vi "GRA_SAPER_RUN.vi"() -> ()   [LabVIEW 2021]
panel:
  out "flag":bool
  out "Czas gry":dbl format="%<%M:%S>t"
  out ".not. x?":bool
  out "Miny":i32
  out "resta":i32
  out "mat17":i32[][](array[numeric])
  out "rozmiar":i32
  in  "cluster3":T1
  in  "Cluster 2":T2
  in  "Cluster 1":T3
  out "licznik":i32[][](array[numeric])
  out "miny":i32[][](array[numeric])
  out "zdjecia":i32[][](array[ring])
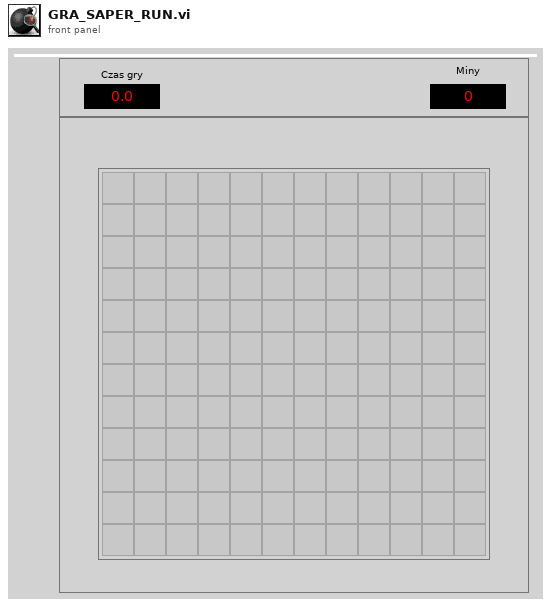
[diagram p1: front panel]
types:
  T1 = cluster{"Boolean 65":bool, "Boolean 66":bool, "Boolean 67":bool, "Boolean 68":bool, "Boolean 69":bool, "Boolean 70":bool, "Boolean 71":bool, "Boolean 72":bool, "Boolean 73":bool, "Boolean 74":bool, "Boolean 75":bool, "Boolean 76":bool, "Boolean 77":bool, "Boolean 78":bool, "Boolean 79":bool, "Boolean 80":bool, "Boolean 81":bool, "Boolean 82":bool, "Boolean 83":bool, "Boolean 84":bool, "Boolean 85":bool, "Boolean 86":bool, "Boolean 87":bool, "Boolean 88":bool, "Boolean 89":bool, "Boolean 90":bool, "Boolean 91":bool, "Boolean 92":bool, "Boolean 93":bool, "Boolean 94":bool, "Boolean 95":bool, "Boolean 96":bool, "Boolean 97":bool, "Boolean 98":bool, "Boolean 99":bool, "Boolean 100":bool, "Boolean 101":bool, "Boolean 102":bool, "Boolean 103":bool, "Boolean 104":bool, "Boolean 105":bool, "Boolean 106":bool, "Boolean 107":bool, "Boolean 108":bool, "Boolean 109":bool, "Boolean 110":bool, "Boolean 111":bool, "Boolean 112":bool, "Boolean 113":bool, "Boolean 114":bool, "Boolean 115":bool, "Boolean 116":bool, "Boolean 117":bool, "Boolean 118":bool, "Boolean 119":bool, "Boolean 120":bool, "Boolean 121":bool, "Boolean 122":bool, "Boolean 123":bool, "Boolean 124":bool, "Boolean 125":bool, "Boolean 126":bool, "Boolean 127":bool, "Boolean 128":bool, "Boolean 129":bool, "Boolean 130":bool, "Boolean 131":bool, "Boolean 132":bool, "Boolean 133":bool, "Boolean 134":bool, "Boolean 135":bool, "Boolean 136":bool, "Boolean 137":bool, "Boolean 138":bool, "Boolean 139":bool, "Boolean 140":bool, "Boolean 141":bool, "Boolean 142":bool, "Boolean 143":bool, "Boolean 144":bool, "Boolean 145":bool, "Boolean 146":bool, "Boolean 147":bool, "Boolean 148":bool, "Boolean 149":bool, "Boolean 150":bool, "Boolean 151":bool, "Boolean 152":bool, "Boolean 153":bool, "Boolean 154":bool, "Boolean 155":bool, "Boolean 156":bool, "Boolean 157":bool, "Boolean 158":bool, "Boolean 159":bool, "Boolean 160":bool, "Boolean 161":bool, "Boolean 162":bool, "Boolean 163":bool, "Boolean 164":bool, "Boolean 165":bool, "Boolean 166":bool, "Boolean 167":bool, "Boolean 168":bool, "Boolean 169":bool, "Boolean 170":bool, "Boolean 171":bool, "Boolean 172":bool, "Boolean 173":bool, "Boolean 174":bool, "Boolean 175":bool, "Boolean 176":bool, "Boolean 177":bool, "Boolean 178":bool, "Boolean 179":bool, "Boolean 180":bool, "Boolean 181":bool, "Boolean 182":bool, "Boolean 183":bool, "Boolean 184":bool, "Boolean 185":bool, "Boolean 186":bool, "Boolean 187":bool, "Boolean 188":bool, "Boolean 189":bool, "Boolean 190":bool, "Boolean 191":bool, "Boolean 192":bool, "Boolean 193":bool, "Boolean 194":bool, "Boolean 195":bool, "Boolean 196":bool, "Boolean 197":bool, "Boolean 198":bool, "Boolean 199":bool, "Boolean 200":bool, "Boolean 201":bool, "Boolean 202":bool, "Boolean 203":bool, "Boolean 204":bool, "Boolean 205":bool, "Boolean 206":bool, "Boolean 207":bool, "Boolean 208":bool}
  T2 = cluster{"Boolean 65":bool, "Boolean 66":bool, "Boolean 67":bool, "Boolean 68":bool, "Boolean 69":bool, "Boolean 70":bool, "Boolean 71":bool, "Boolean 72":bool, "Boolean 77":bool, "Boolean 78":bool, "Boolean 79":bool, "Boolean 80":bool, "Boolean 81":bool, "Boolean 82":bool, "Boolean 83":bool, "Boolean 84":bool, "Boolean 89":bool, "Boolean 90":bool, "Boolean 91":bool, "Boolean 92":bool, "Boolean 93":bool, "Boolean 94":bool, "Boolean 95":bool, "Boolean 96":bool, "Boolean 101":bool, "Boolean 102":bool, "Boolean 103":bool, "Boolean 104":bool, "Boolean 105":bool, "Boolean 106":bool, "Boolean 107":bool, "Boolean 108":bool, "Boolean 113":bool, "Boolean 114":bool, "Boolean 115":bool, "Boolean 116":bool, "Boolean 117":bool, "Boolean 118":bool, "Boolean 119":bool, "Boolean 120":bool, "Boolean 125":bool, "Boolean 126":bool, "Boolean 127":bool, "Boolean 128":bool, "Boolean 129":bool, "Boolean 130":bool, "Boolean 131":bool, "Boolean 132":bool, "Boolean 137":bool, "Boolean 138":bool, "Boolean 139":bool, "Boolean 140":bool, "Boolean 141":bool, "Boolean 142":bool, "Boolean 143":bool, "Boolean 144":bool, "Boolean 149":bool, "Boolean 150":bool, "Boolean 151":bool, "Boolean 152":bool, "Boolean 153":bool, "Boolean 154":bool, "Boolean 155":bool, "Boolean 156":bool}
  T3 = cluster{"Boolean 65":bool, "Boolean 66":bool, "Boolean 67":bool, "Boolean 68":bool, "Boolean 69":bool, "Boolean 70":bool, "Boolean 77":bool, "Boolean 78":bool, "Boolean 79":bool, "Boolean 80":bool, "Boolean 81":bool, "Boolean 82":bool, "Boolean 89":bool, "Boolean 90":bool, "Boolean 91":bool, "Boolean 92":bool, "Boolean 93":bool, "Boolean 94":bool, "Boolean 101":bool, "Boolean 102":bool, "Boolean 103":bool, "Boolean 104":bool, "Boolean 105":bool, "Boolean 106":bool, "Boolean 113":bool, "Boolean 114":bool, "Boolean 115":bool, "Boolean 116":bool, "Boolean 117":bool, "Boolean 118":bool, "Boolean 125":bool, "Boolean 126":bool, "Boolean 127":bool, "Boolean 128":bool, "Boolean 129":bool, "Boolean 130":bool}
  T4 = cluster{"Boolean 6":bool, "Boolean 6":bool, "Boolean 7":bool, "Boolean 8":bool, "Boolean 9":bool, "Boolean 10":bool, "Boolean 11":bool, "Boolean 12":bool, "Boolean 13":bool, "Boolean 14":bool, "Boolean 15":bool, "Boolean 16":bool, "Boolean 17":bool, "Boolean 18":bool, "Boolean 19":bool, "Boolean 20":bool, "Boolean 21":bool, "Boolean 22":bool, "Boolean 23":bool, "Boolean 24":bool, "Boolean 25":bool, "Boolean 26":bool, "Boolean 27":bool, "Boolean 28":bool, "Boolean 29":bool, "Boolean 30":bool, "Boolean 31":bool, "Boolean 32":bool, "Boolean 33":bool, "Boolean 34":bool, "Boolean 35":bool, "Boolean 36":bool, "Boolean 37":bool, "Boolean 38":bool, "Boolean 39":bool, "Boolean 40":bool, "Boolean 41":bool, "Boolean 42":bool, "Boolean 43":bool, "Boolean 44":bool, "Boolean 45":bool, "Boolean 46":bool, "Boolean 47":bool, "Boolean 48":bool, "Boolean 49":bool, "Boolean 50":bool, "Boolean 51":bool, "Boolean 52":bool, "Boolean 53":bool, "Boolean 54":bool, "Boolean 55":bool, "Boolean 56":bool, "Boolean 57":bool, "Boolean 58":bool, "Boolean 59":bool, "Boolean 60":bool, "Boolean 61":bool, "Boolean 62":bool, "Boolean 63":bool, "Boolean 64":bool, "Boolean 65":bool, "Boolean 66":bool, "Boolean 67":bool, "Boolean 68":bool, "Boolean 69":bool, "Boolean 70":bool, "Boolean 71":bool, "Boolean 72":bool, "Boolean 73":bool, "Boolean 74":bool, "Boolean 75":bool, "Boolean 76":bool, "Boolean 77":bool, "Boolean 78":bool, "Boolean 79":bool, "Boolean 80":bool, "Boolean 81":bool, "Boolean 82":bool, "Boolean 83":bool, "Boolean 84":bool, "Boolean 85":bool, "Boolean 86":bool, "Boolean 87":bool, "Boolean 88":bool, "Boolean 89":bool, "Boolean 90":bool, "Boolean 91":bool, "Boolean 92":bool, "Boolean 93":bool, "Boolean 94":bool, "Boolean 95":bool, "Boolean 96":bool, "Boolean 97":bool, "Boolean 98":bool, "Boolean 99":bool, "Boolean 100":bool, "Boolean 101":bool, "Boolean 102":bool, "Boolean 103":bool, "Boolean 104":bool, "Boolean 105":bool, "Boolean 106":bool, "Boolean 107":bool, "Boolean 108":bool, "Boolean 109":bool, "Boolean 110":bool, "Boolean 111":bool, "Boolean 112":bool, "Boolean 113":bool, "Boolean 114":bool, "Boolean 115":bool, "Boolean 116":bool, "Boolean 117":bool, "Boolean 118":bool, "Boolean 119":bool, "Boolean 120":bool, "Boolean 121":bool, "Boolean 122":bool, "Boolean 123":bool, "Boolean 124":bool, "Boolean 125":bool, "Boolean 126":bool, "Boolean 127":bool, "Boolean 128":bool, "Boolean 129":bool, "Boolean 130":bool, "Boolean 131":bool, "Boolean 132":bool, "Boolean 133":bool, "Boolean 134":bool, "Boolean 135":bool, "Boolean 136":bool, "Boolean 137":bool, "Boolean 138":bool, "Boolean 139":bool, "Boolean 140":bool, "Boolean 141":bool, "Boolean 142":bool, "Boolean 143":bool, "Boolean 144":bool, "Boolean 145":bool, "Boolean 146":bool, "Boolean 147":bool, "Boolean 148":bool}
  T5 = cluster{"Boolean 6":bool, "Boolean 6":bool, "Boolean 7":bool, "Boolean 8":bool, "Boolean 9":bool, "Boolean 10":bool, "Boolean 11":bool, "Boolean 12":bool, "Boolean 17":bool, "Boolean 18":bool, "Boolean 19":bool, "Boolean 20":bool, "Boolean 21":bool, "Boolean 22":bool, "Boolean 23":bool, "Boolean 24":bool, "Boolean 29":bool, "Boolean 30":bool, "Boolean 31":bool, "Boolean 32":bool, "Boolean 33":bool, "Boolean 34":bool, "Boolean 35":bool, "Boolean 36":bool, "Boolean 41":bool, "Boolean 42":bool, "Boolean 43":bool, "Boolean 44":bool, "Boolean 45":bool, "Boolean 46":bool, "Boolean 47":bool, "Boolean 48":bool, "Boolean 53":bool, "Boolean 54":bool, "Boolean 55":bool, "Boolean 56":bool, "Boolean 57":bool, "Boolean 58":bool, "Boolean 59":bool, "Boolean 60":bool, "Boolean 65":bool, "Boolean 66":bool, "Boolean 67":bool, "Boolean 68":bool, "Boolean 69":bool, "Boolean 70":bool, "Boolean 71":bool, "Boolean 72":bool, "Boolean 77":bool, "Boolean 78":bool, "Boolean 79":bool, "Boolean 80":bool, "Boolean 81":bool, "Boolean 82":bool, "Boolean 83":bool, "Boolean 84":bool, "Boolean 89":bool, "Boolean 90":bool, "Boolean 91":bool, "Boolean 92":bool, "Boolean 93":bool, "Boolean 94":bool, "Boolean 95":bool, "Boolean 96":bool}
  T6 = cluster{"Boolean 6":bool, "Boolean 6":bool, "Boolean 7":bool, "Boolean 8":bool, "Boolean 9":bool, "Boolean 10":bool, "Boolean 17":bool, "Boolean 18":bool, "Boolean 19":bool, "Boolean 20":bool, "Boolean 21":bool, "Boolean 22":bool, "Boolean 29":bool, "Boolean 30":bool, "Boolean 31":bool, "Boolean 32":bool, "Boolean 33":bool, "Boolean 34":bool, "Boolean 41":bool, "Boolean 42":bool, "Boolean 43":bool, "Boolean 44":bool, "Boolean 45":bool, "Boolean 46":bool, "Boolean 53":bool, "Boolean 54":bool, "Boolean 55":bool, "Boolean 56":bool, "Boolean 57":bool, "Boolean 58":bool, "Boolean 65":bool, "Boolean 66":bool, "Boolean 67":bool, "Boolean 68":bool, "Boolean 69":bool, "Boolean 70":bool}
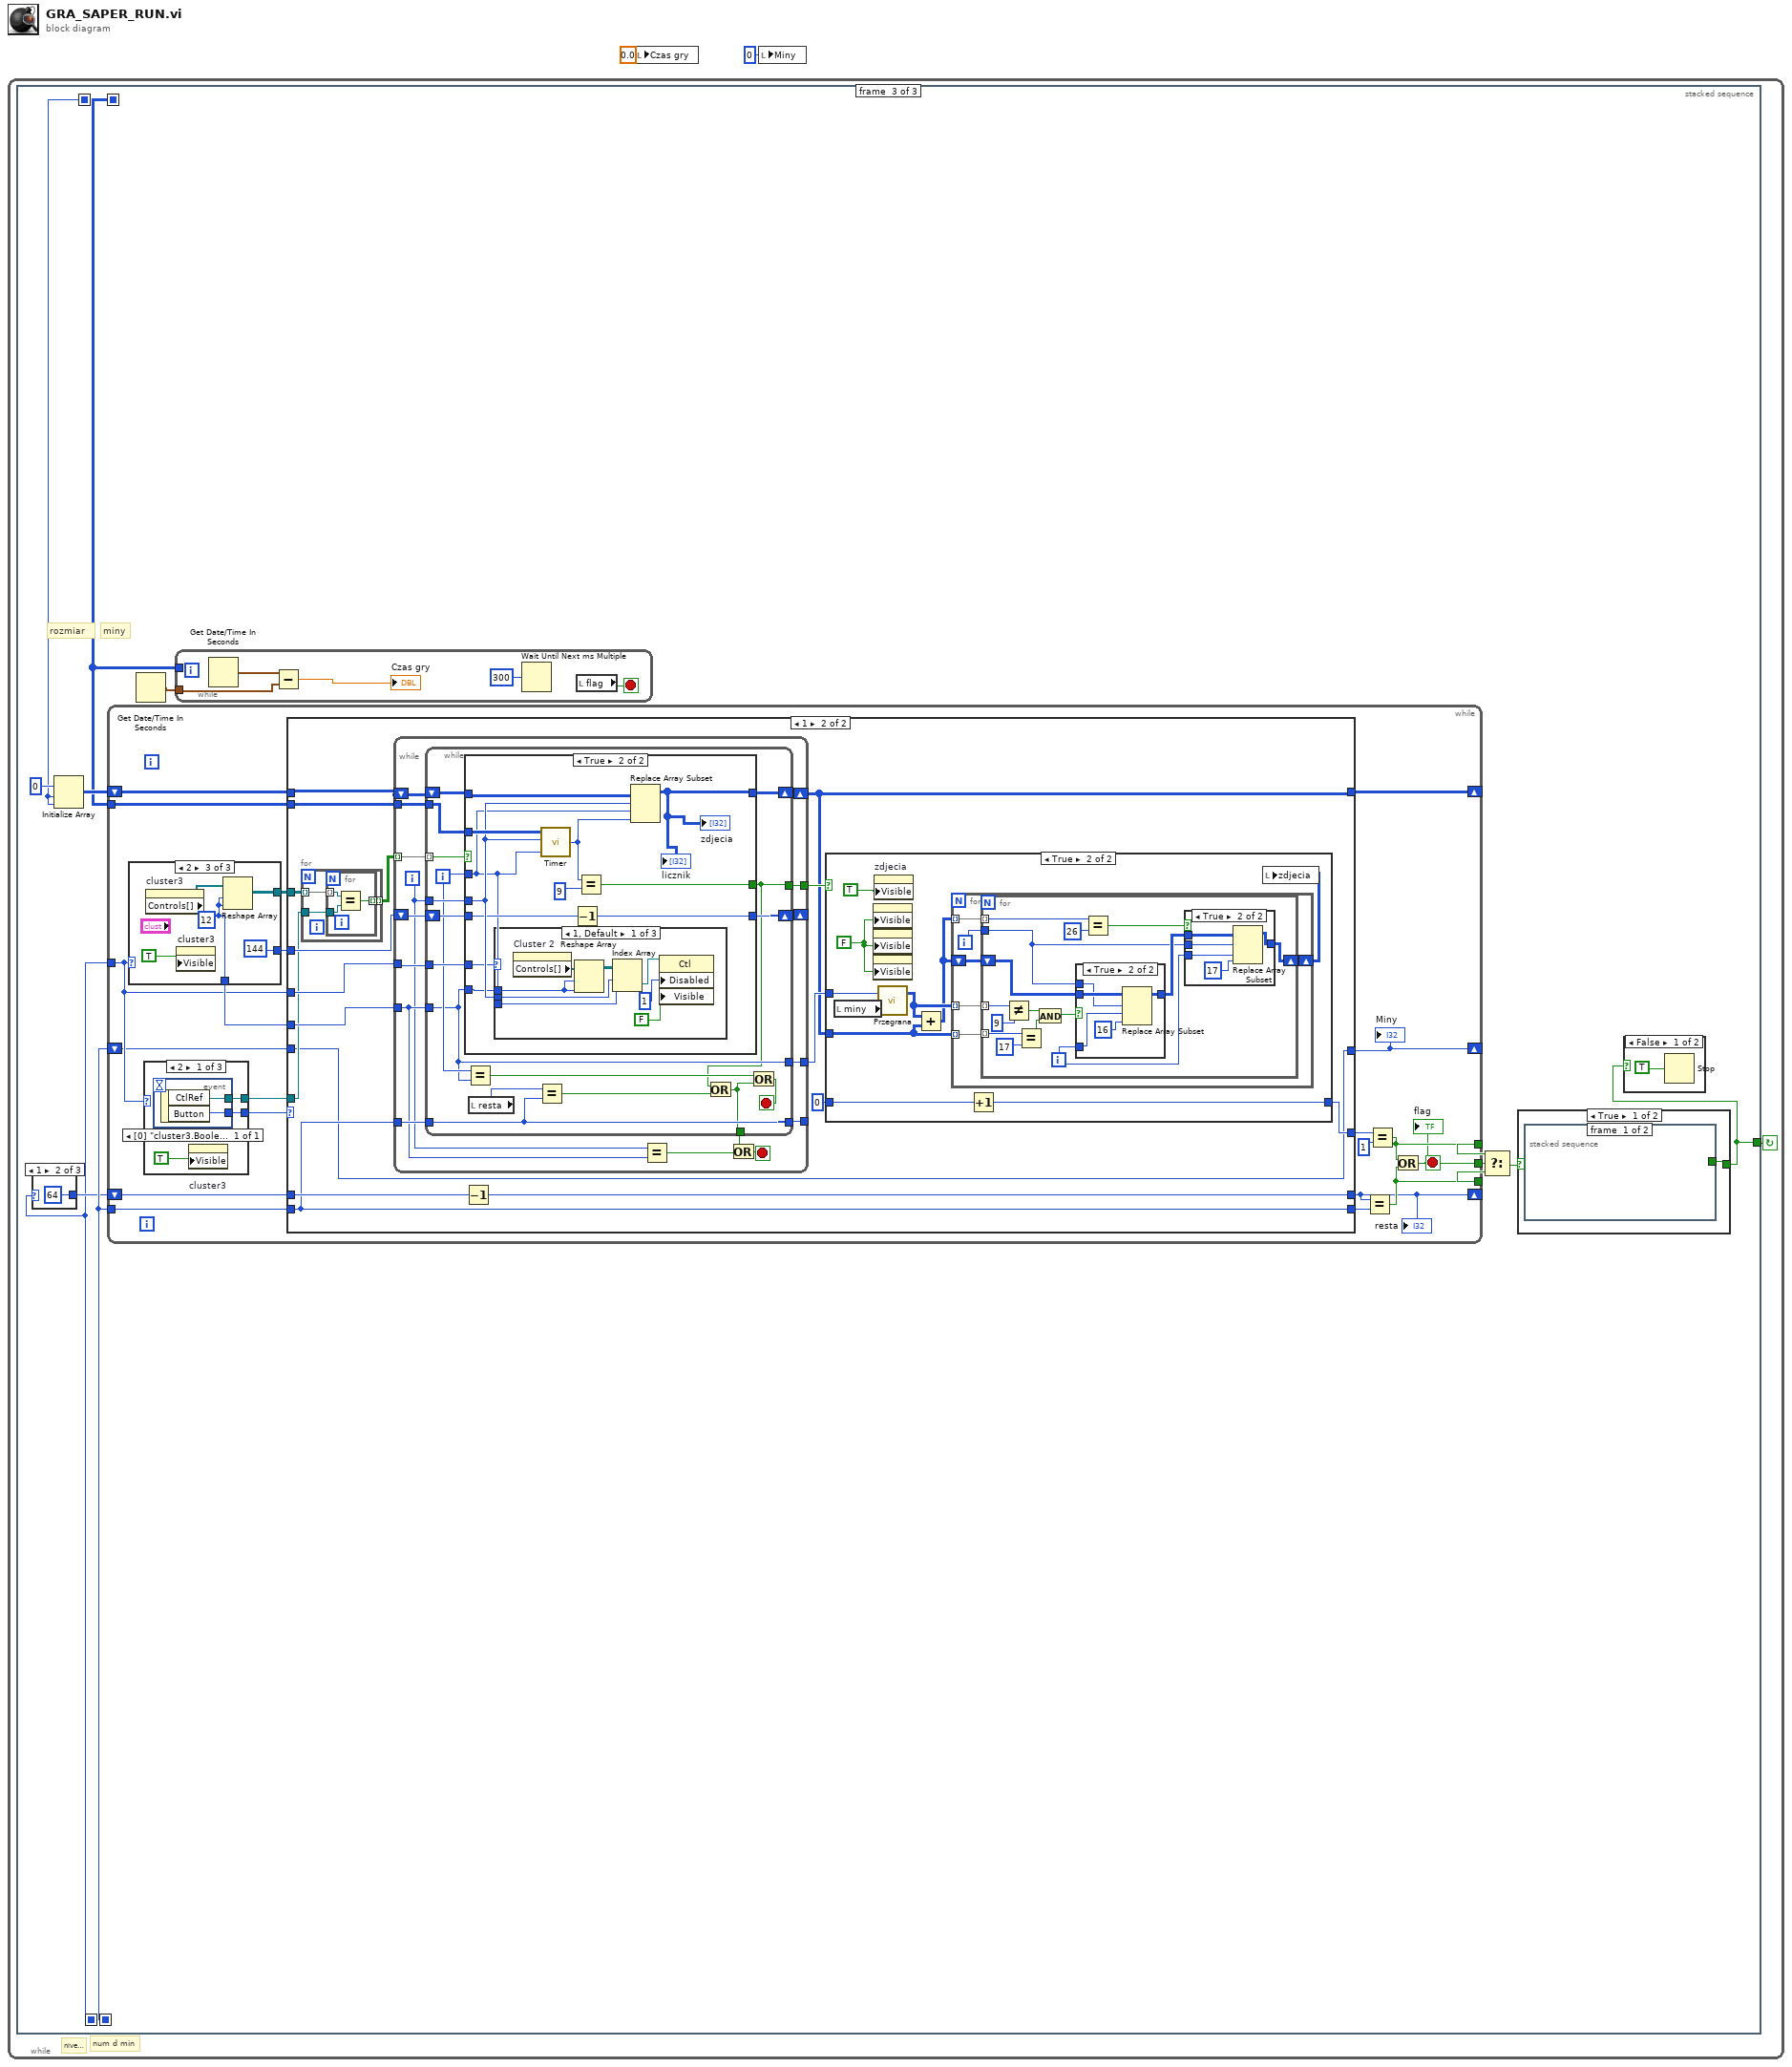
[diagram p0: block diagram]
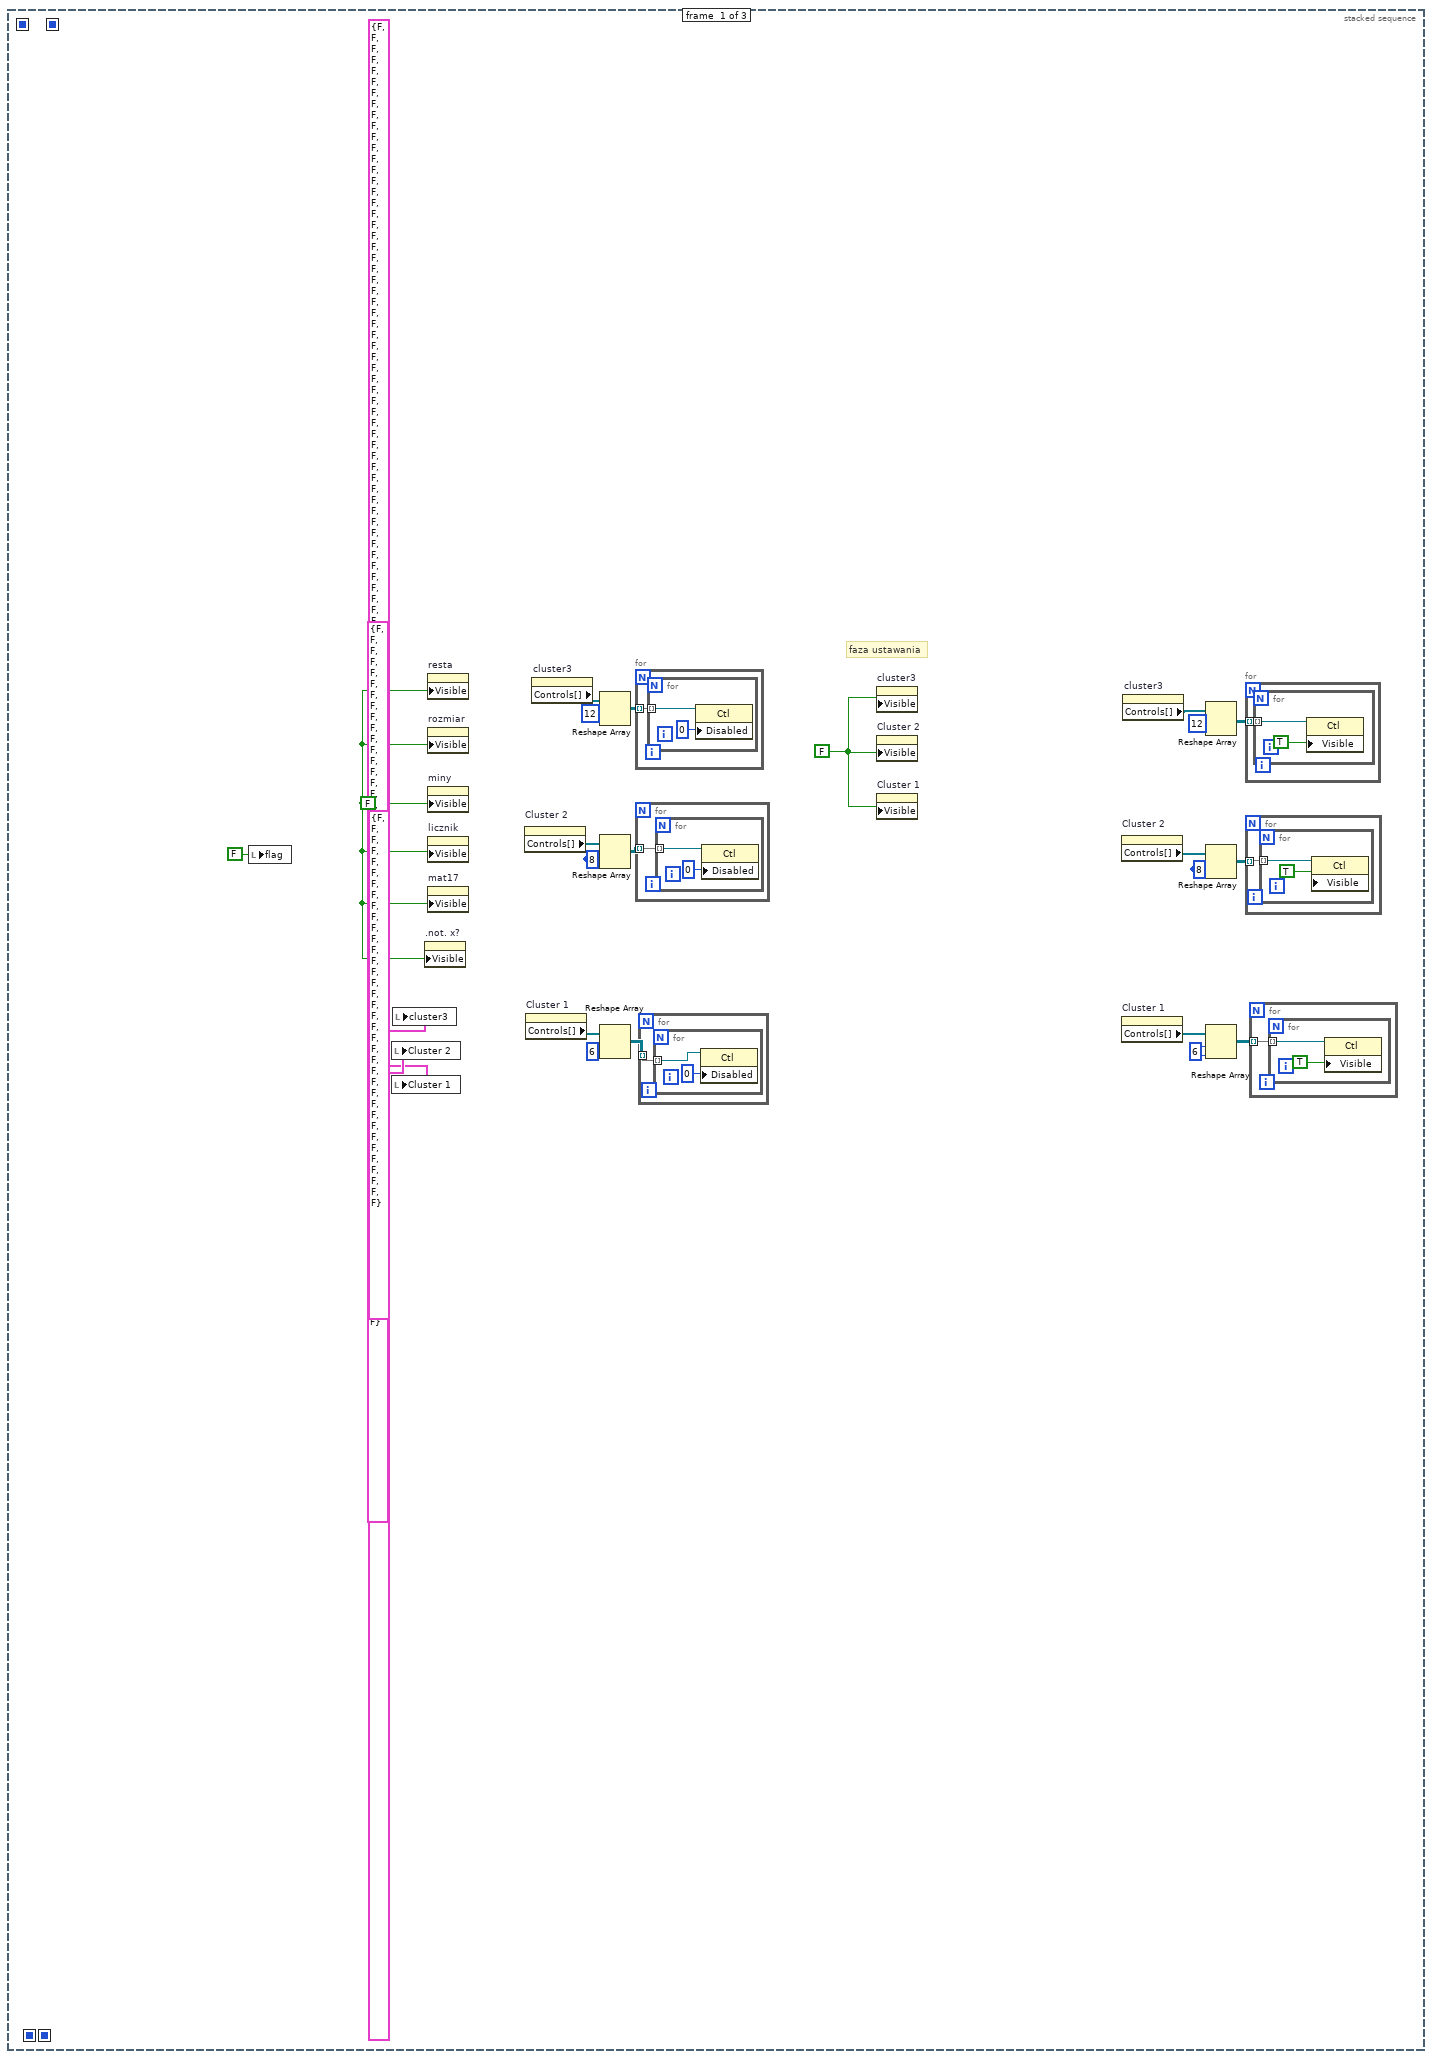
[diagram p2: hidden frame]
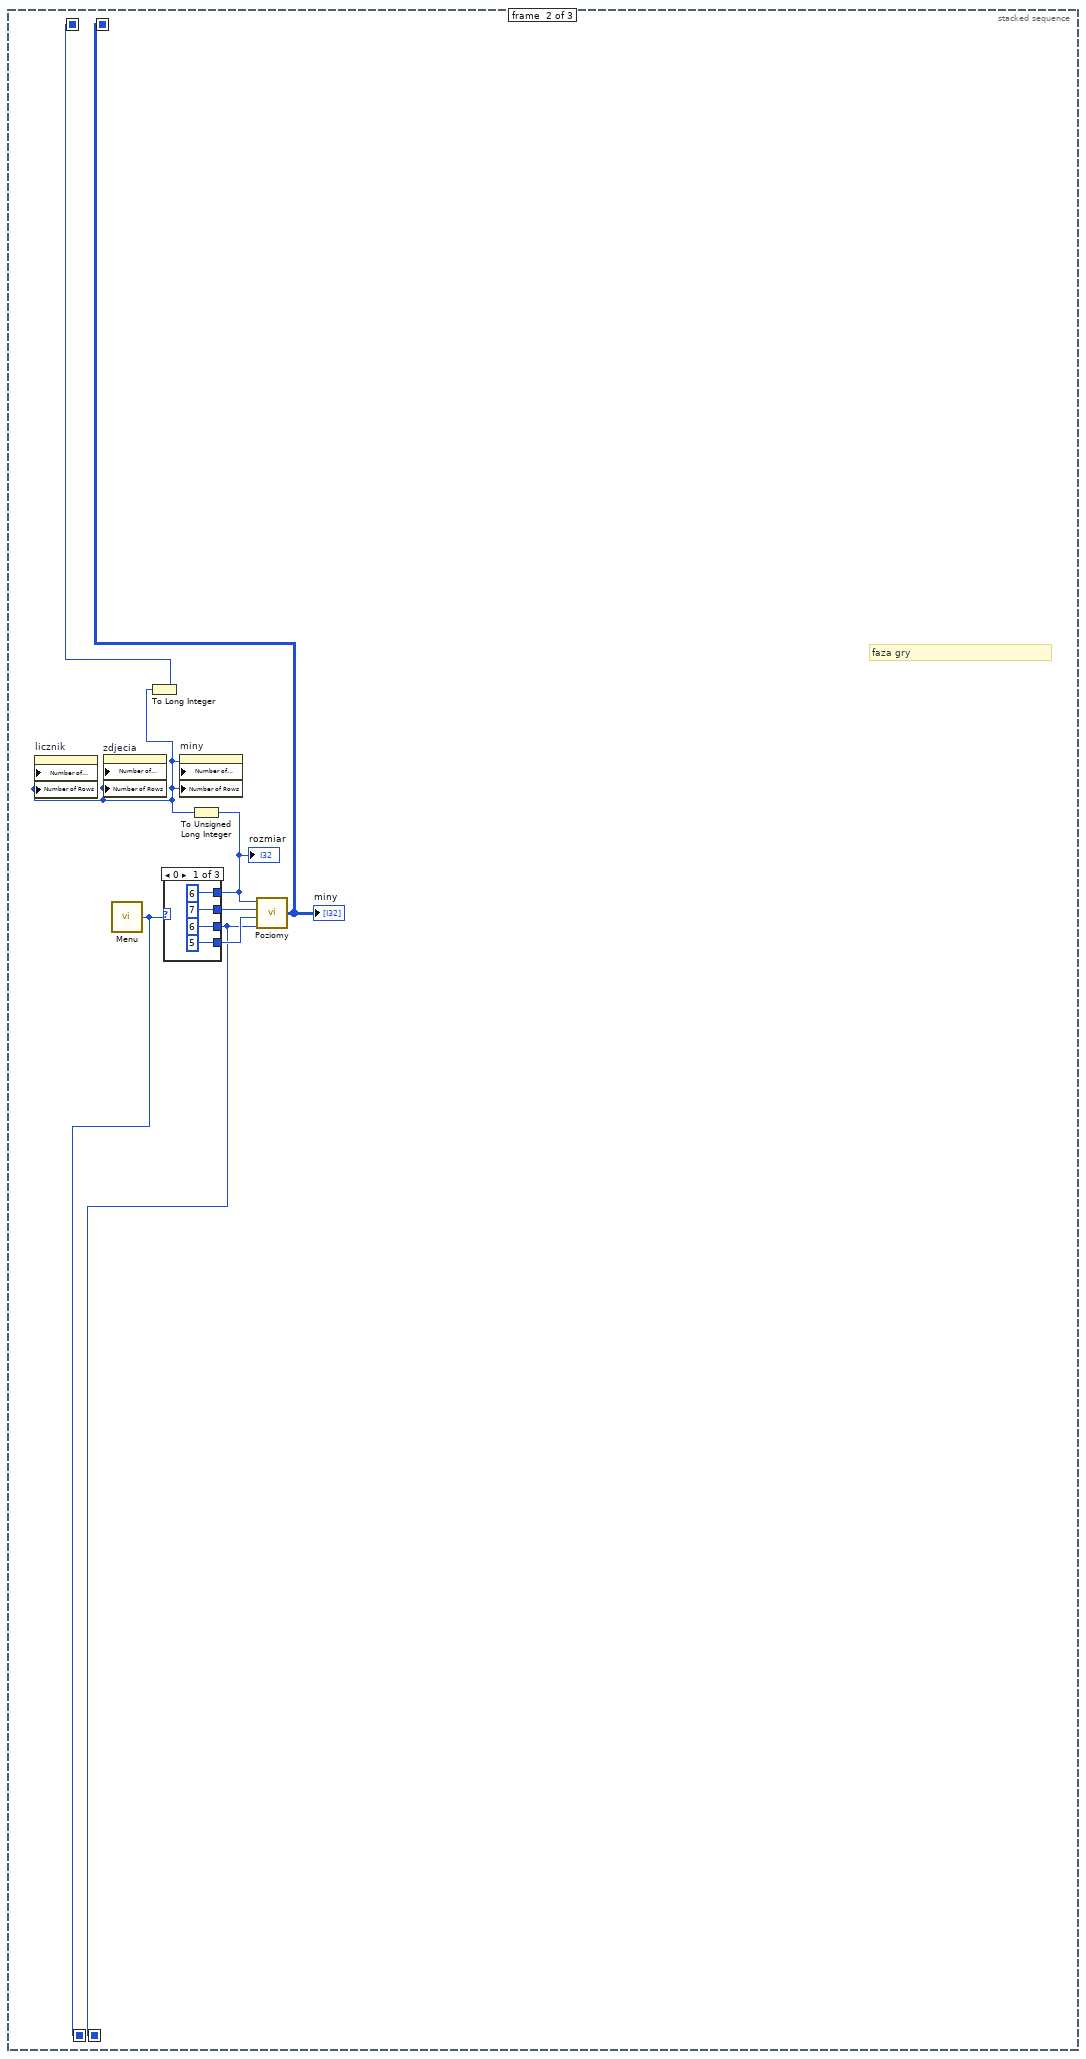
[diagram p3: hidden frame]
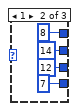
[diagram p4: hidden frame]
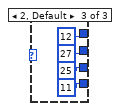
[diagram p5: hidden frame]
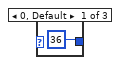
[diagram p6: hidden frame]
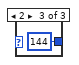
[diagram p7: hidden frame]
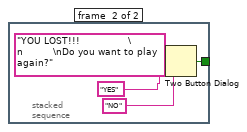
[diagram p8: hidden frame]
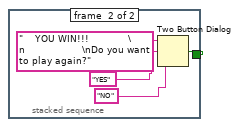
[diagram p10: hidden frame]
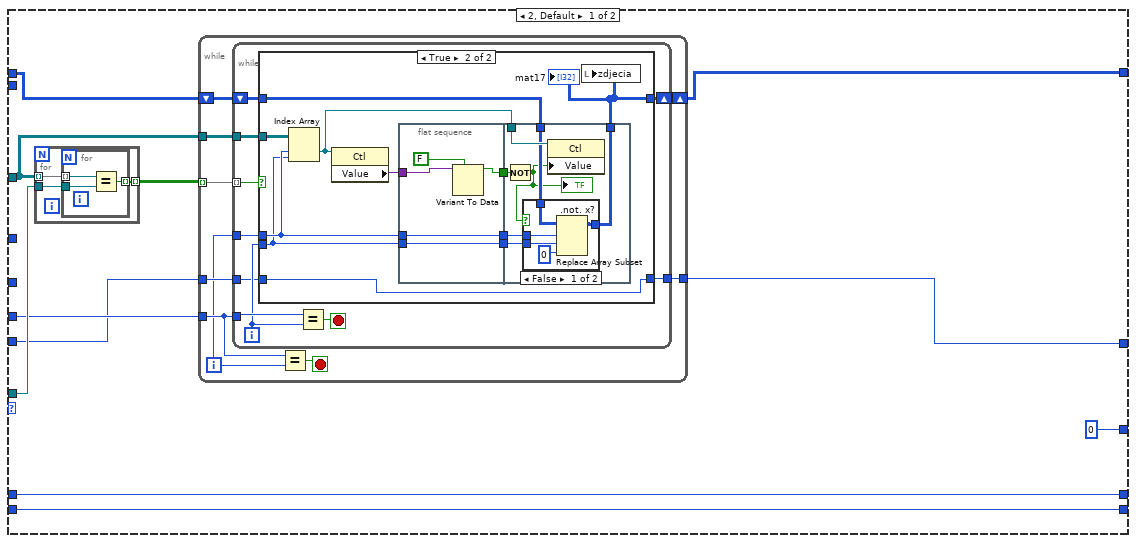
[diagram p11: hidden frame]
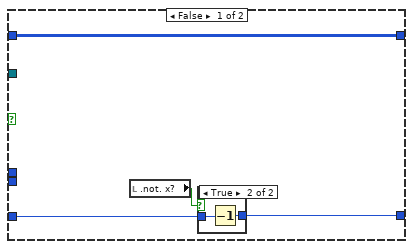
[diagram p12: hidden frame]
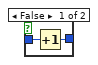
[diagram p13: hidden frame]
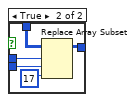
[diagram p14: hidden frame]
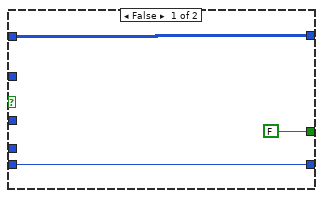
[diagram p18: hidden frame]
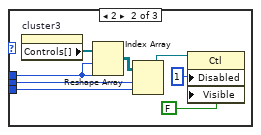
[diagram p19: hidden frame]
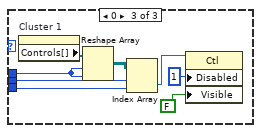
[diagram p20: hidden frame]
diagram:
  n1 = while {
    stop <- w3 continue-if-true
    # "nivepoziom"
    # "num d min"
    # "miny"
    # "rozmiar"
    n2 = stacked-sequence {
      seq-local: [_ w46 _] -> [_ _ w76]
      seq-local: [_ w51 _] -> [_ _ w66]
      seq-local: [_ w49 _] -> [_ _ w72]
      seq-local: [_ w48 _] -> [_ _ w70]
      tunnel: [_ _ w69] -> w3
      frame #0 {
        w5 = FALSE ("Visible")
        w7 = FALSE ("Visible")
        w14 = 12 ("dimension size")
        w11 = 8 ("dimension size")
        w8 = 6 ("dimension size")
        w20 = 12 ("dimension size")
        w23 = 8 ("dimension size")
        w26 = 6 ("dimension size")
        # "faza ustawania"
        n3 = local write "flag"(FALSE ("flag")) -> ()
        n4 = local write "Cluster 2"(T5 {"Boolean 6"=FALSE, "Boolean 6"=FALSE, "Boolean 7"=FALSE, "Boolean 8"=FALSE, "Boolean 9"=FALSE, "Boolean 10"=FALSE, "Boolean 11"=FALSE, "Boolean 12"=FALSE, "Boolean 17"=FALSE, "Boolean 18"=FALSE, "Boolean 19"=FALSE, "Boolean 20"=FALSE, "Boolean 21"=FALSE, "Boolean 22"=FALSE, "Boolean 23"=FALSE, "Boolean 24"=FALSE, "Boolean 29"=FALSE, "Boolean 30"=FALSE, "Boolean 31"=FALSE, "Boolean 32"=FALSE, "Boolean 33"=FALSE, "Boolean 34"=FALSE, "Boolean 35"=FALSE, "Boolean 36"=FALSE, "Boolean 41"=FALSE, "Boolean 42"=FALSE, "Boolean 43"=FALSE, "Boolean 44"=FALSE, "Boolean 45"=FALSE, "Boolean 46"=FALSE, "Boolean 47"=FALSE, "Boolean 48"=FALSE, "Boolean 53"=FALSE, "Boolean 54"=FALSE, "Boolean 55"=FALSE, "Boolean 56"=FALSE, "Boolean 57"=FALSE, "Boolean 58"=FALSE, "Boolean 59"=FALSE, "Boolean 60"=FALSE, "Boolean 65"=FALSE, "Boolean 66"=FALSE, "Boolean 67"=FALSE, "Boolean 68"=FALSE, "Boolean 69"=FALSE, "Boolean 70"=FALSE, "Boolean 71"=FALSE, "Boolean 72"=FALSE, "Boolean 77"=FALSE, "Boolean 78"=FALSE, "Boolean 79"=FALSE, "Boolean 80"=FALSE, "Boolean 81"=FALSE, "Boolean 82"=FALSE, "Boolean 83"=FALSE, "Boolean 84"=FALSE, "Boolean 89"=FALSE, "Boolean 90"=FALSE, "Boolean 91"=FALSE, "Boolean 92"=FALSE, "Boolean 93"=FALSE, "Boolean 94"=FALSE, "Boolean 95"=FALSE, "Boolean 96"=FALSE} ("Cluster 3")) -> ()
        n5 = local write "Cluster 1"(T6 {"Boolean 6"=FALSE, "Boolean 6"=FALSE, "Boolean 7"=FALSE, "Boolean 8"=FALSE, "Boolean 9"=FALSE, "Boolean 10"=FALSE, "Boolean 17"=FALSE, "Boolean 18"=FALSE, "Boolean 19"=FALSE, "Boolean 20"=FALSE, "Boolean 21"=FALSE, "Boolean 22"=FALSE, "Boolean 29"=FALSE, "Boolean 30"=FALSE, "Boolean 31"=FALSE, "Boolean 32"=FALSE, "Boolean 33"=FALSE, "Boolean 34"=FALSE, "Boolean 41"=FALSE, "Boolean 42"=FALSE, "Boolean 43"=FALSE, "Boolean 44"=FALSE, "Boolean 45"=FALSE, "Boolean 46"=FALSE, "Boolean 53"=FALSE, "Boolean 54"=FALSE, "Boolean 55"=FALSE, "Boolean 56"=FALSE, "Boolean 57"=FALSE, "Boolean 58"=FALSE, "Boolean 65"=FALSE, "Boolean 66"=FALSE, "Boolean 67"=FALSE, "Boolean 68"=FALSE, "Boolean 69"=FALSE, "Boolean 70"=FALSE} ("Cluster 1")) -> ()
        n6 = local write "cluster3"(T4 {"Boolean 6"=FALSE, "Boolean 6"=FALSE, "Boolean 7"=FALSE, "Boolean 8"=FALSE, "Boolean 9"=FALSE, "Boolean 10"=FALSE, "Boolean 11"=FALSE, "Boolean 12"=FALSE, "Boolean 13"=FALSE, "Boolean 14"=FALSE, "Boolean 15"=FALSE, "Boolean 16"=FALSE, "Boolean 17"=FALSE, "Boolean 18"=FALSE, "Boolean 19"=FALSE, "Boolean 20"=FALSE, "Boolean 21"=FALSE, "Boolean 22"=FALSE, "Boolean 23"=FALSE, "Boolean 24"=FALSE, "Boolean 25"=FALSE, "Boolean 26"=FALSE, "Boolean 27"=FALSE, "Boolean 28"=FALSE, "Boolean 29"=FALSE, "Boolean 30"=FALSE, "Boolean 31"=FALSE, "Boolean 32"=FALSE, "Boolean 33"=FALSE, "Boolean 34"=FALSE, "Boolean 35"=FALSE, "Boolean 36"=FALSE, "Boolean 37"=FALSE, "Boolean 38"=FALSE, "Boolean 39"=FALSE, "Boolean 40"=FALSE, "Boolean 41"=FALSE, "Boolean 42"=FALSE, "Boolean 43"=FALSE, "Boolean 44"=FALSE, "Boolean 45"=FALSE, "Boolean 46"=FALSE, "Boolean 47"=FALSE, "Boolean 48"=FALSE, "Boolean 49"=FALSE, "Boolean 50"=FALSE, "Boolean 51"=FALSE, "Boolean 52"=FALSE, "Boolean 53"=FALSE, "Boolean 54"=FALSE, "Boolean 55"=FALSE, "Boolean 56"=FALSE, "Boolean 57"=FALSE, "Boolean 58"=FALSE, "Boolean 59"=FALSE, "Boolean 60"=FALSE, "Boolean 61"=FALSE, "Boolean 62"=FALSE, "Boolean 63"=FALSE, "Boolean 64"=FALSE, "Boolean 65"=FALSE, "Boolean 66"=FALSE, "Boolean 67"=FALSE, "Boolean 68"=FALSE, "Boolean 69"=FALSE, "Boolean 70"=FALSE, "Boolean 71"=FALSE, "Boolean 72"=FALSE, "Boolean 73"=FALSE, "Boolean 74"=FALSE, "Boolean 75"=FALSE, "Boolean 76"=FALSE, "Boolean 77"=FALSE, "Boolean 78"=FALSE, "Boolean 79"=FALSE, "Boolean 80"=FALSE, "Boolean 81"=FALSE, "Boolean 82"=FALSE, "Boolean 83"=FALSE, "Boolean 84"=FALSE, "Boolean 85"=FALSE, "Boolean 86"=FALSE, "Boolean 87"=FALSE, "Boolean 88"=FALSE, "Boolean 89"=FALSE, "Boolean 90"=FALSE, "Boolean 91"=FALSE, "Boolean 92"=FALSE, "Boolean 93"=FALSE, "Boolean 94"=FALSE, "Boolean 95"=FALSE, "Boolean 96"=FALSE, "Boolean 97"=FALSE, "Boolean 98"=FALSE, "Boolean 99"=FALSE, "Boolean 100"=FALSE, "Boolean 101"=FALSE, "Boolean 102"=FALSE, "Boolean 103"=FALSE, "Boolean 104"=FALSE, "Boolean 105"=FALSE, "Boolean 106"=FALSE, "Boolean 107"=FALSE, "Boolean 108"=FALSE, "Boolean 109"=FALSE, "Boolean 110"=FALSE, "Boolean 111"=FALSE, "Boolean 112"=FALSE, "Boolean 113"=FALSE, "Boolean 114"=FALSE, "Boolean 115"=FALSE, "Boolean 116"=FALSE, "Boolean 117"=FALSE, "Boolean 118"=FALSE, "Boolean 119"=FALSE, "Boolean 120"=FALSE, "Boolean 121"=FALSE, "Boolean 122"=FALSE, "Boolean 123"=FALSE, "Boolean 124"=FALSE, "Boolean 125"=FALSE, "Boolean 126"=FALSE, "Boolean 127"=FALSE, "Boolean 128"=FALSE, "Boolean 129"=FALSE, "Boolean 130"=FALSE, "Boolean 131"=FALSE, "Boolean 132"=FALSE, "Boolean 133"=FALSE, "Boolean 134"=FALSE, "Boolean 135"=FALSE, "Boolean 136"=FALSE, "Boolean 137"=FALSE, "Boolean 138"=FALSE, "Boolean 139"=FALSE, "Boolean 140"=FALSE, "Boolean 141"=FALSE, "Boolean 142"=FALSE, "Boolean 143"=FALSE, "Boolean 144"=FALSE, "Boolean 145"=FALSE, "Boolean 146"=FALSE, "Boolean 147"=FALSE, "Boolean 148"=FALSE} ("Cluster 4")) -> ()
        n7 = property on=".not. x?" class="Bool (strict)"("Visible"=w5) -> ()  [unwired: 2 in, 2 out]
        n8 = property on="resta" class="DigNum (strict)"("Visible"=w5) -> ()  [unwired: 2 in, 2 out]
        n9 = property on="rozmiar" class="DigNum (strict)"("Visible"=w5) -> ()  [unwired: 2 in, 2 out]
        n10 = property on="miny" class="Arr (strict)"("Visible"=w5) -> ()  [unwired: 2 in, 2 out]
        n11 = property on="licznik" class="Arr (strict)"("Visible"=w5) -> ()  [unwired: 2 in, 2 out]
        n12 = property on="mat17" class="Arr (strict)"("Visible"=w5) -> ()  [unwired: 2 in, 2 out]
        n13 = property on="Cluster 2" class="Clust (strict)"() -> ("Controls[]"=w22:refnum<vi>[])  [unwired: 2 in, 2 out]
        n14 = property on="Cluster 1" class="Clust (strict)"() -> ("Controls[]"=w27:refnum<vi>[])  [unwired: 2 in, 2 out]
        n15 = property on="cluster3" class="Clust (strict)"() -> ("Controls[]"=w19:refnum<vi>[])  [unwired: 2 in, 2 out]
        n16 = Reshape Array(w19, w20, w20) -> (w21:refnum<vi>[][])
        n17 = Reshape Array(w22, w23, w23) -> (w24:refnum<vi>[][])
        n18 = Reshape Array(w27, w26, w26) -> (w25:refnum<vi>[][])
        n19 = for {
          tunnel: w21 -> [w37] mode=indexing
          n20 = for {
            tunnel: w37 -> [w39] mode=indexing
            n21 = property class="Ctl"(reference=w39, "Disabled"=u8 0) -> ()  [unwired: 1 in, 2 out]
          }
        }
        n22 = for {
          tunnel: w24 -> [w40] mode=indexing
          n23 = for {
            tunnel: w40 -> [w42] mode=indexing
            n24 = property class="Ctl"(reference=w42, "Disabled"=u8 0) -> ()  [unwired: 1 in, 2 out]
          }
        }
        n25 = for {
          tunnel: w25 -> [w43] mode=indexing
          n26 = for {
            tunnel: w43 -> [w45] mode=indexing
            n27 = property class="Ctl"(reference=w45, "Disabled"=u8 0) -> ()  [unwired: 1 in, 2 out]
          }
        }
        n28 = property on="cluster3" class="Clust (strict)"("Visible"=w7) -> ()  [unwired: 2 in, 2 out]
        n29 = property on="Cluster 2" class="Clust (strict)"("Visible"=w7) -> ()  [unwired: 2 in, 2 out]
        n30 = property on="Cluster 1" class="Clust (strict)"("Visible"=w7) -> ()  [unwired: 2 in, 2 out]
        n31 = property on="Cluster 2" class="Clust (strict)"() -> ("Controls[]"=w12:refnum<vi>[])  [unwired: 2 in, 2 out]
        n32 = property on="Cluster 1" class="Clust (strict)"() -> ("Controls[]"=w6:refnum<vi>[])  [unwired: 2 in, 2 out]
        n33 = property on="cluster3" class="Clust (strict)"() -> ("Controls[]"=w15:refnum<vi>[])  [unwired: 2 in, 2 out]
        n34 = Reshape Array(w15, w14, w14) -> (w13:refnum<vi>[][])
        n35 = Reshape Array(w12, w11, w11) -> (w10:refnum<vi>[][])
        n36 = Reshape Array(w6, w8, w8) -> (w9:refnum<vi>[][])
        n37 = for {
          tunnel: w13 -> [w28] mode=indexing
          n38 = for {
            tunnel: w28 -> [w30] mode=indexing
            n39 = property class="Ctl"(reference=w30, "Visible"=TRUE) -> ()  [unwired: 1 in, 2 out]
          }
        }
        n40 = for {
          tunnel: w10 -> [w31] mode=indexing
          n41 = for {
            tunnel: w31 -> [w33] mode=indexing
            n42 = property class="Ctl"(reference=w33, "Visible"=TRUE) -> ()  [unwired: 1 in, 2 out]
          }
        }
        n43 = for {
          tunnel: w9 -> [w34] mode=indexing
          n44 = for {
            tunnel: w34 -> [w36] mode=indexing
            n45 = property class="Ctl"(reference=w36, "Visible"=TRUE) -> ()  [unwired: 1 in, 2 out]
          }
        }
      }
      frame #1 {
        # "faza gry"
        n46 = call "Menu.vi"() -> ("result"=w48:i32)
        n47 = case shown="0" w48 {
          tunnel: [6 8 12] -> w50
          tunnel: [7 14 27] -> w53
          tunnel: [6 12 25] -> w49
          tunnel: [5 7 11] -> w52
          frame 0 {
          }
          frame 1 {
          }
          frame 2, Default {
          }
        }
        "rozmiar" <- w50
        n48 = To Unsigned Long Integer(number=w50) -> (unsigned 32bit integer=w47:u32)
        n49 = property on="licznik" class="Arr (strict)"("Number of Columns"=w47, "Number of Rows"=w47) -> ()  [unwired: 2 in, 2 out]
        n50 = property on="zdjecia" class="Arr (strict)"("Number of Columns"=w47, "Number of Rows"=w47) -> ()  [unwired: 2 in, 2 out]
        n51 = To Long Integer(number=w47) -> (32bit integer=w46:i32)
        n52 = property on="miny" class="Arr (strict)"("Number of Columns"=w47, "Number of Rows"=w47) -> ()  [unwired: 2 in, 2 out]
        n53 = call "Poziomy.vi"("Miny"=w49, "cons"=w52, "Mina nr1"=w53, "Rozmiar"=w50) -> ("Array"=w51:i32[][])
        "miny" <- w51
      }
      frame #2 {
        n54 = case shown="1" w70 {
          tunnel: [36 ("dimension size") 64 ("dimension size") 144 ("dimension size")] -> w71
          frame 0, Default {
          }
          frame 1 {
          }
          frame 2 {
          }
        }
        n55 = Initialize Array(0 ("element"), w76, w76) -> (w77:i32[][])
        n56 = while {
          tunnel: w66 -> [w116]
          tunnel: w70 -> [w108]
          shift-right: [w106] -> _
          shift-left: w77 -> [w115]
          tunnel: w72 -> [w113]
          tunnel: [w100] -> w68
          tunnel: [w101] -> w75
          tunnel: [w102] -> w74
          shift-right: [w99] -> _
          shift-left: w71 -> [w104]
          shift-right: [w97] -> _
          shift-left: w72 -> [w98]
          stop <- w100 stop-if-true
          n57 = case shown="2" w108 {
            tunnel: [w349 w354 w359] -> w114
            tunnel: [36 ("dimension size") 64 ("element") 144] -> w112
            tunnel: [w348 w353 w358] -> w107
            frame 0, Default {
              w349 = 6 ("dimension size")
              n58 = property on="Cluster 1" class="Clust (strict)"() -> ("Controls[]"=w350:refnum<vi>[])  [unwired: 2 in, 2 out]
              n59 = property on="Cluster 1" class="Clust (strict)"("Visible"=TRUE) -> ()  [unwired: 2 in, 2 out]
              n60 = Reshape Array(w350, w349, w349) -> (w348:refnum<vi>[][])
            }
            frame 1 {
              w354 = 8 ("element")
              n61 = property on="Cluster 2" class="Clust (strict)"() -> ("Controls[]"=w355:refnum<vi>[])  [unwired: 2 in, 2 out]
              n62 = property on="Cluster 2" class="Clust (strict)"("Visible"=TRUE) -> ()  [unwired: 2 in, 2 out]
              n63 = Reshape Array(w355, w354, w354) -> (w353:refnum<vi>[][])
            }
            frame 2 {
              w359 = 12 ("element")
              n64 = property on="cluster3" class="Clust (strict)"() -> ("Controls[]"=w360:refnum<vi>[])  [unwired: 2 in, 2 out]
              n65 = property on="cluster3" class="Clust (strict)"("Visible"=TRUE) -> ()  [unwired: 2 in, 2 out]
              n66 = Reshape Array(w360, w359, w359) -> (w358:refnum<vi>[][])
            }
          }
          n67 = case shown="2" w108 {
            tunnel: [w335 w340 w345] -> w110
            tunnel: [w334 w339 w343] -> w109
            frame 2 {
              n68 = event shown="[0] \"cluster3.Boolean 65\", \"cluster3.Boolean 66\", \"cluster3.Boolean 67\", \"cluster3.Boolean 68\", \"cluster3.Boolean 69\", \"cluster3.Boolean 70\", \"cluster3.Boolean 71\", \"cluster3.Boolean 72\", \"cluster3.Boolean 73\", \"cluster3.Boolean 74\", \"cluster3.Boolean 75\", \"cluster3.Boolean 76\", \"cluster3.Boolean 77\", \"cluster3.Boolean 78\", \"cluster3.Boolean 79\", \"cluster3.Boolean 80\", \"cluster3.Boolean 81\", \"cluster3.Boolean 82\", \"cluster3.Boolean 83\", \"cluster3.Boolean 84\", \"cluster3.Boolean 85\", \"cluster3.Boolean 86\", \"cluster3.Boolean 87\", \"cluster3.Boolean 88\", \"cluster3.Boolean 89\", \"cluster3.Boolean 90\", \"cluster3.Boolean 91\", \"cluster3.Boolean 92\", \"cluster3.Boolean 93\", \"cluster3.Boolean 94\", \"cluster3.Boolean 95\", \"cluster3.Boolean 96\", \"cluster3.Boolean 97\", \"cluster3.Boolean 98\", \"cluster3.Boolean 99\", \"cluster3.Boolean 100\", \"cluster3.Boolean 101\", \"cluster3.Boolean 102\", \"cluster3.Boolean 103\", \"cluster3.Boolean 104\", \"cluster3.Boolean 105\", \"cluster3.Boolean 106\", \"cluster3.Boolean 107\", \"cluster3.Boolean 108\", \"cluster3.Boolean 109\", \"cluster3.Boolean 110\", \"cluster3.Boolean 111\", \"cluster3.Boolean 112\", \"cluster3.Boolean 113\", \"cluster3.Boolean 114\", \"cluster3.Boolean 115\", \"cluster3.Boolean 116\", \"cluster3.Boolean 117\", \"cluster3.Boolean 118\", \"cluster3.Boolean 119\", \"cluster3.Boolean 120\", \"cluster3.Boolean 121\", \"cluster3.Boolean 122\", \"cluster3.Boolean 123\", \"cluster3.Boolean 124\", \"cluster3.Boolean 125\", \"cluster3.Boolean 126\", \"cluster3.Boolean 127\", \"cluster3.Boolean 128\", \"cluster3.Boolean 129\", \"cluster3.Boolean 130\", \"cluster3.Boolean 131\", \"cluster3.Boolean 132\", \"cluster3.Boolean 133\", \"cluster3.Boolean 134\", \"cluster3.Boolean 135\", \"cluster3.Boolean 136\", \"cluster3.Boolean 137\", \"cluster3.Boolean 138\", \"cluster3.Boolean 139\", \"cluster3.Boolean 140\", \"cluster3.Boolean 141\", \"cluster3.Boolean 142\", \"cluster3.Boolean 143\", \"cluster3.Boolean 144\", \"cluster3.Boolean 145\", \"cluster3.Boolean 146\", \"cluster3.Boolean 147\", \"cluster3.Boolean 148\", \"cluster3.Boolean 149\", \"cluster3.Boolean 150\", \"cluster3.Boolean 151\", \"cluster3.Boolean 152\", \"cluster3.Boolean 153\", \"cluster3.Boolean 154\", \"cluster3.Boolean 155\", \"cluster3.Boolean 156\", \"cluster3.Boolean 157\", \"cluster3.Boolean 158\", \"cluster3.Boolean 159\", \"cluster3.Boolean 160\", \"cluster3.Boolean 161\", \"cluster3.Boolean 162\", \"cluster3.Boolean 163\", \"cluster3.Boolean 164\", \"cluster3.Boolean 165\", \"cluster3.Boolean 166\", \"cluster3.Boolean 167\", \"cluster3.Boolean 168\", \"cluster3.Boolean 169\", \"cluster3.Boolean 170\", \"cluster3.Boolean 171\", \"cluster3.Boolean 172\", \"cluster3.Boolean 173\", \"cluster3.Boolean 174\", \"cluster3.Boolean 175\", \"cluster3.Boolean 176\", \"cluster3.Boolean 177\", \"cluster3.Boolean 178\", \"cluster3.Boolean 179\", \"cluster3.Boolean 180\", \"cluster3.Boolean 181\", \"cluster3.Boolean 182\", \"cluster3.Boolean 183\", \"cluster3.Boolean 184\", \"cluster3.Boolean 185\", \"cluster3.Boolean 186\", \"cluster3.Boolean 187\", \"cluster3.Boolean 188\", \"cluster3.Boolean 189\", \"cluster3.Boolean 190\", \"cluster3.Boolean 191\", \"cluster3.Boolean 192\", \"cluster3.Boolean 193\", \"cluster3.Boolean 194\", \"cluster3.Boolean 195\", \"cluster3.Boolean 196\", \"cluster3.Boolean 197\", \"cluster3.Boolean 198\", \"cluster3.Boolean 199\", \"cluster3.Boolean 200\", \"cluster3.Boolean 201\", \"cluster3.Boolean 202\", \"cluster3.Boolean 203\", \"cluster3.Boolean 204\", \"cluster3.Boolean 205\", \"cluster3.Boolean 206\", \"cluster3.Boolean 207\", \"cluster3.Boolean 208\": Mouse Down" {
                selector: _ -> [_]
                dyn-events: _ -> [_]
                timeout: _ -> [_]
                tunnel: [w336] -> w335
                tunnel: [w337] -> w334
                event "cluster3.Boolean 65", "cluster3.Boolean 66", "cluster3.Boolean 67", "cluster3.Boolean 68", "cluster3.Boolean 69", "cluster3.Boolean 70", "cluster3.Boolean 71", "cluster3.Boolean 72", "cluster3.Boolean 73", "cluster3.Boolean 74", "cluster3.Boolean 75", "cluster3.Boolean 76", "cluster3.Boolean 77", "cluster3.Boolean 78", "cluster3.Boolean 79", "cluster3.Boolean 80", "cluster3.Boolean 81", "cluster3.Boolean 82", "cluster3.Boolean 83", "cluster3.Boolean 84", "cluster3.Boolean 85", "cluster3.Boolean 86", "cluster3.Boolean 87", "cluster3.Boolean 88", "cluster3.Boolean 89", "cluster3.Boolean 90", "cluster3.Boolean 91", "cluster3.Boolean 92", "cluster3.Boolean 93", "cluster3.Boolean 94", "cluster3.Boolean 95", "cluster3.Boolean 96", "cluster3.Boolean 97", "cluster3.Boolean 98", "cluster3.Boolean 99", "cluster3.Boolean 100", "cluster3.Boolean 101", "cluster3.Boolean 102", "cluster3.Boolean 103", "cluster3.Boolean 104", "cluster3.Boolean 105", "cluster3.Boolean 106", "cluster3.Boolean 107", "cluster3.Boolean 108", "cluster3.Boolean 109", "cluster3.Boolean 110", "cluster3.Boolean 111", "cluster3.Boolean 112", "cluster3.Boolean 113", "cluster3.Boolean 114", "cluster3.Boolean 115", "cluster3.Boolean 116", "cluster3.Boolean 117", "cluster3.Boolean 118", "cluster3.Boolean 119", "cluster3.Boolean 120", "cluster3.Boolean 121", "cluster3.Boolean 122", "cluster3.Boolean 123", "cluster3.Boolean 124", "cluster3.Boolean 125", "cluster3.Boolean 126", "cluster3.Boolean 127", "cluster3.Boolean 128", "cluster3.Boolean 129", "cluster3.Boolean 130", "cluster3.Boolean 131", "cluster3.Boolean 132", "cluster3.Boolean 133", "cluster3.Boolean 134", "cluster3.Boolean 135", "cluster3.Boolean 136", "cluster3.Boolean 137", "cluster3.Boolean 138", "cluster3.Boolean 139", "cluster3.Boolean 140", "cluster3.Boolean 141", "cluster3.Boolean 142", "cluster3.Boolean 143", "cluster3.Boolean 144", "cluster3.Boolean 145", "cluster3.Boolean 146", "cluster3.Boolean 147", "cluster3.Boolean 148", "cluster3.Boolean 149", "cluster3.Boolean 150", "cluster3.Boolean 151", "cluster3.Boolean 152", "cluster3.Boolean 153", "cluster3.Boolean 154", "cluster3.Boolean 155", "cluster3.Boolean 156", "cluster3.Boolean 157", "cluster3.Boolean 158", "cluster3.Boolean 159", "cluster3.Boolean 160", "cluster3.Boolean 161", "cluster3.Boolean 162", "cluster3.Boolean 163", "cluster3.Boolean 164", "cluster3.Boolean 165", "cluster3.Boolean 166", "cluster3.Boolean 167", "cluster3.Boolean 168", "cluster3.Boolean 169", "cluster3.Boolean 170", "cluster3.Boolean 171", "cluster3.Boolean 172", "cluster3.Boolean 173", "cluster3.Boolean 174", "cluster3.Boolean 175", "cluster3.Boolean 176", "cluster3.Boolean 177", "cluster3.Boolean 178", "cluster3.Boolean 179", "cluster3.Boolean 180", "cluster3.Boolean 181", "cluster3.Boolean 182", "cluster3.Boolean 183", "cluster3.Boolean 184", "cluster3.Boolean 185", "cluster3.Boolean 186", "cluster3.Boolean 187", "cluster3.Boolean 188", "cluster3.Boolean 189", "cluster3.Boolean 190", "cluster3.Boolean 191", "cluster3.Boolean 192", "cluster3.Boolean 193", "cluster3.Boolean 194", "cluster3.Boolean 195", "cluster3.Boolean 196", "cluster3.Boolean 197", "cluster3.Boolean 198", "cluster3.Boolean 199", "cluster3.Boolean 200", "cluster3.Boolean 201", "cluster3.Boolean 202", "cluster3.Boolean 203", "cluster3.Boolean 204", "cluster3.Boolean 205", "cluster3.Boolean 206", "cluster3.Boolean 207", "cluster3.Boolean 208": Mouse Down {
                  n69 = event-data() -> ("CtlRef"=w337:refnum<vi>, "Button"=w336:u16)  [unwired: 1 in]
                }
              }
              n70 = property on="cluster3" class="Clust (strict)"("Visible"=TRUE) -> ()  [unwired: 2 in, 2 out]
            }
            frame 1, Default {
              n71 = event shown="[0] \"Cluster 2.Boolean 65\", \"Cluster 2.Boolean 66\", \"Cluster 2.Boolean 67\", \"Cluster 2.Boolean 68\", \"Cluster 2.Boolean 69\", \"Cluster 2.Boolean 70\", \"Cluster 2.Boolean 71\", \"Cluster 2.Boolean 72\", \"Cluster 2.Boolean 77\", \"Cluster 2.Boolean 78\", \"Cluster 2.Boolean 79\", \"Cluster 2.Boolean 80\", \"Cluster 2.Boolean 81\", \"Cluster 2.Boolean 82\", \"Cluster 2.Boolean 83\", \"Cluster 2.Boolean 84\", \"Cluster 2.Boolean 89\", \"Cluster 2.Boolean 90\", \"Cluster 2.Boolean 91\", \"Cluster 2.Boolean 92\", \"Cluster 2.Boolean 93\", \"Cluster 2.Boolean 94\", \"Cluster 2.Boolean 95\", \"Cluster 2.Boolean 96\", \"Cluster 2.Boolean 101\", \"Cluster 2.Boolean 102\", \"Cluster 2.Boolean 103\", \"Cluster 2.Boolean 104\", \"Cluster 2.Boolean 105\", \"Cluster 2.Boolean 106\", \"Cluster 2.Boolean 107\", \"Cluster 2.Boolean 108\", \"Cluster 2.Boolean 113\", \"Cluster 2.Boolean 114\", \"Cluster 2.Boolean 115\", \"Cluster 2.Boolean 116\", \"Cluster 2.Boolean 117\", \"Cluster 2.Boolean 118\", \"Cluster 2.Boolean 119\", \"Cluster 2.Boolean 120\", \"Cluster 2.Boolean 125\", \"Cluster 2.Boolean 126\", \"Cluster 2.Boolean 127\", \"Cluster 2.Boolean 128\", \"Cluster 2.Boolean 129\", \"Cluster 2.Boolean 130\", \"Cluster 2.Boolean 131\", \"Cluster 2.Boolean 132\", \"Cluster 2.Boolean 137\", \"Cluster 2.Boolean 138\", \"Cluster 2.Boolean 139\", \"Cluster 2.Boolean 140\", \"Cluster 2.Boolean 141\", \"Cluster 2.Boolean 142\", \"Cluster 2.Boolean 143\", \"Cluster 2.Boolean 144\", \"Cluster 2.Boolean 149\", \"Cluster 2.Boolean 150\", \"Cluster 2.Boolean 151\", \"Cluster 2.Boolean 152\", \"Cluster 2.Boolean 153\", \"Cluster 2.Boolean 154\", \"Cluster 2.Boolean 155\", \"Cluster 2.Boolean 156\": Mouse Down" {
                selector: _ -> [_]
                dyn-events: _ -> [_]
                timeout: _ -> [_]
                tunnel: [w342] -> w340
                tunnel: [w341] -> w339
                event "Cluster 2.Boolean 65", "Cluster 2.Boolean 66", "Cluster 2.Boolean 67", "Cluster 2.Boolean 68", "Cluster 2.Boolean 69", "Cluster 2.Boolean 70", "Cluster 2.Boolean 71", "Cluster 2.Boolean 72", "Cluster 2.Boolean 77", "Cluster 2.Boolean 78", "Cluster 2.Boolean 79", "Cluster 2.Boolean 80", "Cluster 2.Boolean 81", "Cluster 2.Boolean 82", "Cluster 2.Boolean 83", "Cluster 2.Boolean 84", "Cluster 2.Boolean 89", "Cluster 2.Boolean 90", "Cluster 2.Boolean 91", "Cluster 2.Boolean 92", "Cluster 2.Boolean 93", "Cluster 2.Boolean 94", "Cluster 2.Boolean 95", "Cluster 2.Boolean 96", "Cluster 2.Boolean 101", "Cluster 2.Boolean 102", "Cluster 2.Boolean 103", "Cluster 2.Boolean 104", "Cluster 2.Boolean 105", "Cluster 2.Boolean 106", "Cluster 2.Boolean 107", "Cluster 2.Boolean 108", "Cluster 2.Boolean 113", "Cluster 2.Boolean 114", "Cluster 2.Boolean 115", "Cluster 2.Boolean 116", "Cluster 2.Boolean 117", "Cluster 2.Boolean 118", "Cluster 2.Boolean 119", "Cluster 2.Boolean 120", "Cluster 2.Boolean 125", "Cluster 2.Boolean 126", "Cluster 2.Boolean 127", "Cluster 2.Boolean 128", "Cluster 2.Boolean 129", "Cluster 2.Boolean 130", "Cluster 2.Boolean 131", "Cluster 2.Boolean 132", "Cluster 2.Boolean 137", "Cluster 2.Boolean 138", "Cluster 2.Boolean 139", "Cluster 2.Boolean 140", "Cluster 2.Boolean 141", "Cluster 2.Boolean 142", "Cluster 2.Boolean 143", "Cluster 2.Boolean 144", "Cluster 2.Boolean 149", "Cluster 2.Boolean 150", "Cluster 2.Boolean 151", "Cluster 2.Boolean 152", "Cluster 2.Boolean 153", "Cluster 2.Boolean 154", "Cluster 2.Boolean 155", "Cluster 2.Boolean 156": Mouse Down {
                  n72 = event-data() -> ("CtlRef"=w341:refnum<vi>, "Button"=w342:u16)  [unwired: 1 in]
                }
              }
              n73 = property on="Cluster 2" class="Clust (strict)"("Visible"=TRUE) -> ()  [unwired: 2 in, 2 out]
            }
            frame 0 {
              n74 = event shown="[0] \"Cluster 1.Boolean 65\", \"Cluster 1.Boolean 66\", \"Cluster 1.Boolean 67\", \"Cluster 1.Boolean 68\", \"Cluster 1.Boolean 69\", \"Cluster 1.Boolean 70\", \"Cluster 1.Boolean 77\", \"Cluster 1.Boolean 78\", \"Cluster 1.Boolean 80\", \"Cluster 1.Boolean 79\", \"Cluster 1.Boolean 81\", \"Cluster 1.Boolean 82\", \"Cluster 1.Boolean 89\", \"Cluster 1.Boolean 90\", \"Cluster 1.Boolean 91\", \"Cluster 1.Boolean 92\", \"Cluster 1.Boolean 93\", \"Cluster 1.Boolean 94\", \"Cluster 1.Boolean 101\", \"Cluster 1.Boolean 102\", \"Cluster 1.Boolean 103\", \"Cluster 1.Boolean 104\", \"Cluster 1.Boolean 105\", \"Cluster 1.Boolean 106\", \"Cluster 1.Boolean 113\", \"Cluster 1.Boolean 114\", \"Cluster 1.Boolean 115\", \"Cluster 1.Boolean 116\", \"Cluster 1.Boolean 117\", \"Cluster 1.Boolean 118\", \"Cluster 1.Boolean 125\", \"Cluster 1.Boolean 126\", \"Cluster 1.Boolean 127\", \"Cluster 1.Boolean 128\", \"Cluster 1.Boolean 129\", \"Cluster 1.Boolean 130\": Mouse Down" {
                selector: _ -> [_]
                dyn-events: _ -> [_]
                timeout: _ -> [_]
                tunnel: [w346] -> w345
                tunnel: [w347] -> w343
                event "Cluster 1.Boolean 65", "Cluster 1.Boolean 66", "Cluster 1.Boolean 67", "Cluster 1.Boolean 68", "Cluster 1.Boolean 69", "Cluster 1.Boolean 70", "Cluster 1.Boolean 77", "Cluster 1.Boolean 78", "Cluster 1.Boolean 80", "Cluster 1.Boolean 79", "Cluster 1.Boolean 81", "Cluster 1.Boolean 82", "Cluster 1.Boolean 89", "Cluster 1.Boolean 90", "Cluster 1.Boolean 91", "Cluster 1.Boolean 92", "Cluster 1.Boolean 93", "Cluster 1.Boolean 94", "Cluster 1.Boolean 101", "Cluster 1.Boolean 102", "Cluster 1.Boolean 103", "Cluster 1.Boolean 104", "Cluster 1.Boolean 105", "Cluster 1.Boolean 106", "Cluster 1.Boolean 113", "Cluster 1.Boolean 114", "Cluster 1.Boolean 115", "Cluster 1.Boolean 116", "Cluster 1.Boolean 117", "Cluster 1.Boolean 118", "Cluster 1.Boolean 125", "Cluster 1.Boolean 126", "Cluster 1.Boolean 127", "Cluster 1.Boolean 128", "Cluster 1.Boolean 129", "Cluster 1.Boolean 130": Mouse Down {
                  n75 = event-data() -> ("CtlRef"=w347:refnum<vi>, "Button"=w346:u16)  [unwired: 1 in]
                }
              }
              n76 = property on="Cluster 1" class="Clust (strict)"("Visible"=TRUE) -> ()  [unwired: 2 in, 2 out]
            }
          }
          n77 = case shown="1" w110 {
            tunnel: w116 -> [_ w210]
            tunnel: w108 -> [_ w209]
            tunnel: w115 -> [w122 w208]
            tunnel: [w121 w201] -> w106
            tunnel: w114 -> [w123 w207]
            tunnel: w113 -> [w119 w195]
            tunnel: [0 w204] -> w105
            tunnel: w112 -> [_ w199]
            tunnel: w109 -> [w127 w197]
            tunnel: w107 -> [w125 w198]
            tunnel: [w119 w195] -> w103
            tunnel: [w120 w200] -> w99
            tunnel: w104 -> [w120 w196]
            tunnel: [w117 w194] -> w97
            tunnel: w98 -> [w118 w194]
            frame 2, Default {
              n78 = for {
                tunnel: w127 -> [w190]
                tunnel: w125 -> [w189] mode=indexing
                tunnel: [w188] -> w126 mode=indexing
                n79 = for {
                  tunnel: w190 -> [w193]
                  tunnel: w189 -> [w192] mode=indexing
                  tunnel: [w191] -> w188 mode=indexing
                  n80 = Equal?(x=w192, y=w193) -> (x = y?=w191:bool)
                }
              }
              n81 = while {
                tunnel: w126 -> [w136] mode=indexing
                shift-right: [w131] -> w121
                shift-left: w122 -> [w135]
                tunnel: w125 -> [w134]
                tunnel: w123 -> [w133]
                tunnel: w118 -> [w130]
                tunnel: [w128] -> w117
                i -> [w129]
                stop <- w132 stop-if-true
                n82 = while {
                  tunnel: w136 -> [w146] mode=indexing
                  tunnel: w129 -> [w144]
                  shift-right: [w143] -> w131
                  shift-left: w135 -> [w145]
                  tunnel: w134 -> [w142]
                  tunnel: w133 -> [w141]
                  tunnel: w130 -> [w139]
                  tunnel: [w138] -> w128
                  i -> [w140]
                  stop <- w137 stop-if-true
                  n83 = case shown="True" w146 {
                    tunnel: w145 -> [w150 w161]
                    tunnel: w144 -> [_ w159]
                    tunnel: [w150 w158] -> w143
                    tunnel: w142 -> [_ w165]
                    tunnel: w140 -> [_ w156]
                    tunnel: w139 -> [w148 w155]
                    tunnel: [w147 w155] -> w138
                    frame False {
                      n84 = local read ".not. x?"() -> (w149:bool)
                      n85 = case shown="True" w149 {
                        tunnel: [w152 w154] -> w147
                        tunnel: w148 -> [w151 w153]
                        frame False {
                          n86 = Increment(x=w151) -> (x+1=w152:i32)
                        }
                        frame True {
                          n87 = Decrement(x=w153) -> (x-1=w154:i32)
                        }
                      }
                    }
                    frame True {
                      n88 = Index Array(array=w165, index (row)=w159, index (col)=w156) -> (element=w162:refnum<vi>)
                      n89 = property class="Ctl"(reference=w162) -> ("Value"=w163:variant)  [unwired: 1 in, 2 out]
                      n90 = flat-sequence {
                        tunnel: w163 -> [w170]
                        tunnel: [w166] -> w164
                        tunnel: [w169] -> w160
                        tunnel: w159 -> [w169]
                        tunnel: w156 -> [w167]
                        tunnel: [w167] -> w157
                        tunnel: w164 -> [w177]
                        tunnel: w162 -> [w176]
                        tunnel: w161 -> [w175]
                        tunnel: w160 -> [w174]
                        tunnel: [w173] -> w158
                        tunnel: w157 -> [w171]
                        frame #0 {
                          n91 = Variant To Data(type=FALSE ("Visible"), Variant=w170) -> (data=w166:bool)  [unwired: 1 in, 1 out]
                        }
                        frame #1 {
                          n92 = Not(x=w177) -> (.not. x?=w172:bool)
                          ".not. x?" <- w172
                          n93 = case shown="False" w172 {
                            tunnel: w175 -> [w182 w187]
                            tunnel: w174 -> [w180 w186]
                            tunnel: [w181 w184] -> w173
                            tunnel: w171 -> [w178 w185]
                            frame False {
                              n94 = Replace Array Subset(array=w182, new element=0 ("new element/subarray"), index (row)=w180, index (col)=w178) -> (w181:i32[][])
                            }
                            frame True {
                              n95 = Replace Array Subset(array=w187, new element=17 ("new element/subarray"), index (row)=w186, index (col)=w185) -> (w184:i32[][])
                            }
                          }
                          n96 = property class="Ctl"(reference=w176, "Value"=w172) -> ()  [unwired: 1 in, 2 out]
                        }
                      }
                      n97 = local write "zdjecia"(w158) -> ()
                      "mat17" <- w158
                    }
                  }
                  n98 = Equal?(x=w141, y=w140) -> (x = y?=w137:bool)
                }
                n99 = Equal?(x=w133, y=w129) -> (x = y?=w132:bool)
              }
            }
            frame 1 {
              n100 = for {
                tunnel: w197 -> [w213]
                tunnel: [w212] -> w202 mode=indexing
                tunnel: w198 -> [w211] mode=indexing
                n101 = for {
                  tunnel: w211 -> [w214] mode=indexing
                  tunnel: w213 -> [w216]
                  tunnel: [w215] -> w212 mode=indexing
                  n102 = Equal?(x=w214, y=w216) -> (x = y?=w215:bool)
                }
              }
              n103 = while {
                shift-right: [w275] -> w201
                shift-left: w208 -> [w276]
                tunnel: w210 -> [w274]
                tunnel: w207 -> [w268]
                tunnel: w209 -> [w273]
                tunnel: w195 -> [w272]
                shift-right: [w269] -> _
                shift-left: w199 -> [w271]
                tunnel: [w270] -> _
                tunnel: [w264] -> w206
                tunnel: [w263] -> w205
                tunnel: w202 -> [w262] mode=indexing
                i -> [w261]
                stop <- w266 stop-if-true
                n104 = while {
                  shift-right: [w289] -> w275
                  shift-left: w276 -> [w293]
                  tunnel: w261 -> [w292]
                  tunnel: w274 -> [w291]
                  tunnel: w268 -> [w278]
                  tunnel: w273 -> [w290]
                  tunnel: w272 -> [w283]
                  shift-right: [w288] -> w269
                  shift-left: w271 -> [w287]
                  tunnel: [w283] -> w270
                  tunnel: [w281] -> w265
                  tunnel: [w278] -> w263
                  tunnel: [w277] -> w264
                  tunnel: w262 -> [w279] mode=indexing
                  i -> [w286]
                  stop <- w285 stop-if-true
                  n105 = case shown="True" w279 {
                    tunnel: [w296 w297] -> w289
                    tunnel: w293 -> [w296 w308]
                    tunnel: w292 -> [_ w304]
                    tunnel: w286 -> [_ w299]
                    tunnel: w291 -> [_ w307]
                    tunnel: w278 -> [_ w302]
                    tunnel: w290 -> [_ w303]
                    tunnel: [FALSE w300] -> w277
                    tunnel: w287 -> [w294 w301]
                    tunnel: [w294 w298] -> w288
                    frame False {
                    }
                    frame True {
                      n106 = case shown="1, Default" w303 {
                        tunnel: w304 -> [w315 w322 w329]
                        tunnel: w299 -> [w314 w324 w332]
                        tunnel: w302 -> [w312 w321 w328]
                        frame 1, Default {
                          n107 = property on="Cluster 2" class="Clust (strict)"() -> ("Controls[]"=w311:refnum<vi>[])  [unwired: 2 in, 2 out]
                          n108 = Reshape Array(w311, w312, w312) -> (w310:refnum<vi>[][])
                          n109 = Index Array(array=w310, index (row)=w315, index (col)=w314) -> (element=w316:refnum<vi>)
                          n110 = property class="Ctl"(reference=w316, "Disabled"=u8 1, "Visible"=FALSE) -> ()  [unwired: 1 in, 2 out]
                        }
                        frame 2 {
                          n111 = property on="cluster3" class="Clust (strict)"() -> ("Controls[]"=w319:refnum<vi>[])  [unwired: 2 in, 2 out]
                          n112 = Reshape Array(w319, w321, w321) -> (w318:refnum<vi>[][])
                          n113 = Index Array(array=w318, index (row)=w322, index (col)=w324) -> (element=w323:refnum<vi>)
                          n114 = property class="Ctl"(reference=w323, "Disabled"=u8 1, "Visible"=FALSE) -> ()  [unwired: 1 in, 2 out]
                        }
                        frame 0 {
                          n115 = property on="Cluster 1" class="Clust (strict)"() -> ("Controls[]"=w327:refnum<vi>[])  [unwired: 2 in, 2 out]
                          n116 = Reshape Array(w327, w328, w328) -> (w326:refnum<vi>[][])
                          n117 = Index Array(array=w326, index (row)=w329, index (col)=w332) -> (element=w331:refnum<vi>)
                          n118 = property class="Ctl"(reference=w331, "Disabled"=u8 1, "Visible"=FALSE) -> ()  [unwired: 1 in, 2 out]
                        }
                      }
                      n119 = call "Timer.vi"("Kolumny"=w299, "rzedy"=w304, "Array"=w307) -> ("timer"=w305:i32)
                      n120 = Decrement(x=w301) -> (x-1=w298:i32)
                      n121 = Equal?(x=w305, y=9) -> (x = y?=w300:bool)
                      n122 = Replace Array Subset(array=w308, new element=w305, index (row)=w304, index (col)=w299) -> (w297:i32[][])
                      "licznik" <- w297
                      "zdjecia" <- w297
                    }
                  }
                  n123 = Equal?(x=w286, y=w278) -> (x = y?=w280:bool)
                  n124 = local read "resta"() -> (w284:i32)
                  n125 = Equal?(x=w284, y=w283) -> (x = y?=w282:bool)
                  n126 = Or(x=w277, y=w282) -> (x .or. y?=w281:bool)
                  n127 = Or(x=w280, y=w281) -> (x .or. y?=w285:bool)
                }
                n128 = Equal?(x=w261, y=w268) -> (x = y?=w267:bool)
                n129 = Or(x=w267, y=w265) -> (x .or. y?=w266:bool)
              }
              n130 = Decrement(x=w196) -> (x-1=w200:i32)
              n131 = case shown="True" w206 {
                tunnel: w205 -> [_ w223]
                tunnel: 0 -> [w217 w227]
                tunnel: [w217 w226] -> w204
                tunnel: w201 -> [_ w220]
                frame False {
                }
                frame True {
                  w225 = FALSE
                  n132 = local read "miny"() -> (w222:i32[][])
                  n133 = property on="Cluster 1" class="Clust (strict)"("Visible"=w225) -> ()  [unwired: 2 in, 2 out]
                  n134 = property on="cluster3" class="Clust (strict)"("Visible"=w225) -> ()  [unwired: 2 in, 2 out]
                  n135 = property on="Cluster 2" class="Clust (strict)"("Visible"=w225) -> ()  [unwired: 2 in, 2 out]
                  n136 = property on="zdjecia" class="Arr (strict)"("Visible"=TRUE) -> ()  [unwired: 2 in, 2 out]
                  n137 = call "Przegrana.vi"("miny"=w222, "Rozmiar"=w223) -> ("Array 2"=w219:i32[][])  [unwired: 1 in]
                  n138 = Add(x=w219, y=w220) -> (x+y=w218:i32[][])
                  n139 = for {
                    tunnel: w220 -> [w233] mode=indexing
                    tunnel: w219 -> [w232] mode=indexing
                    shift-right: [w229] -> w221
                    shift-left: w218 -> [w231]
                    tunnel: w218 -> [w228] mode=indexing
                    i -> [w230]
                    n140 = for {
                      tunnel: w233 -> [w245] mode=indexing
                      tunnel: w232 -> [w247] mode=indexing
                      tunnel: w230 -> [w235]
                      shift-right: [w236] -> w229
                      shift-left: w231 -> [w248]
                      tunnel: w228 -> [w240] mode=indexing
                      i -> [w234]
                      n141 = Not Equal?(x=w247, y=9) -> (x != y?=w243:bool)
                      n142 = Equal?(x=w245, y=17) -> (x = y?=w242:bool)
                      n143 = And(x=w243, y=w242) -> (x .and. y?=w241:bool)
                      n144 = case shown="True" w241 {
                        tunnel: w248 -> [w255 w260]
                        tunnel: w234 -> [_ w259]
                        tunnel: w235 -> [_ w258]
                        tunnel: [w255 w257] -> w237
                        frame False {
                        }
                        frame True {
                          n145 = Replace Array Subset(array=w260, new element=16, index (row)=w258, index (col)=w259) -> (w257:i32[][])
                        }
                      }
                      n146 = Equal?(x=w240, y=26) -> (x = y?=w238:bool)
                      n147 = case shown="True" w238 {
                        tunnel: w237 -> [w249 w254]
                        tunnel: [w249 w250] -> w236
                        tunnel: w235 -> [_ w253]
                        tunnel: w234 -> [_ w252]
                        frame False {
                        }
                        frame True {
                          n148 = Replace Array Subset(array=w254, new element=17 ("element"), index (row)=w253, index (col)=w252) -> (w250:i32[][])
                        }
                      }
                    }
                  }
                  n149 = Increment(x=w227) -> (x+1=w226:i32)
                  n150 = local write "zdjecia"(w221) -> ()
                }
              }
            }
          }
          "resta" <- w99
          "Miny" <- w97
          n151 = Equal?(x=w99, y=w103) -> (x = y?=w101:bool)
          n152 = Equal?(x=w105, y=1) -> (x = y?=w102:bool)
          n153 = Or(x=w102, y=w101) -> (x .or. y?=w100:bool)
          "flag" <- w100
        }
        n154 = Get Date/Time In Seconds() -> (seconds since 1Jan1904=w67:timestamp)
        n155 = while {
          tunnel: w67 -> [w81]
          tunnel: w66 -> [_]
          stop <- w83 stop-if-true
          n156 = Get Date/Time In Seconds() -> (seconds since 1Jan1904=w82:timestamp)
          n157 = Subtract(x=w82, y=w81) -> (x-y=→"Czas gry":dbl)
          n158 = Wait Until Next ms Multiple(millisecond multiple=u32 300) -> ()  [unwired: 1 out]
          n159 = local read "flag"() -> (w83:bool)
        }
        n160 = Select(t=w74, s=w68, f=w75) -> (s? t:f=w73:bool)
        n161 = case shown="True" w73 {
          tunnel: [w87 w92] -> w69
          frame True {
            n162 = stacked-sequence {
              tunnel: [_ w88] -> w87
              frame #0 {
              }
              frame #1 {
                n163 = Two Button Dialog(message="YOU LOST!!!                \n          \nDo you want to play again?", 1:"NO" ("button name (\"OK\")"), 2:"YES" ("button name (\"OK\")")) -> (T button?=w88:bool)
              }
            }
          }
          frame False {
            n164 = stacked-sequence {
              tunnel: [_ w95] -> w92
              frame #0 {
              }
              frame #1 {
                n165 = Two Button Dialog(message="    YOU WIN!!!             \n                   \nDo you want to play again?", 1:"NO" ("button name (\"OK\")"), 2:"YES" ("button name (\"OK\")")) -> (T button?=w95:bool)
              }
            }
          }
        }
        n166 = case shown="False" w69 {
          frame False {
            n167 = Stop(stop? (T)=TRUE) -> ()
          }
          frame True {
          }
        }
      }
    }
  }
  n168 = local write "Czas gry"(0.0 ("Tiempo")) -> ()
  n169 = local write "Miny"(0 ("Minas")) -> ()
